vi "Configure Instrument.vi"(8 "error in (no error)":errorcluster, 11 "Instrument.Aerotech":refnum<class "Instrument.Aerotech.lvclass">) -> (0 "error out":errorcluster, 3 "Instrument.Aerotech out":refnum<class "Instrument.Aerotech.lvclass">)   [LabVIEW 2016, in "Instrument.Aerotech.lvclass"]
uses:
  Instrument.Aerotech.lvclass
  <userlib>/LevyLab/Levylab Instruments/Instrument Types/Optical Delay Line/Instrument.OpticalDelayLine.lvclass
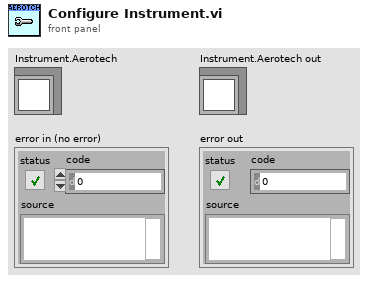
[diagram p1: front panel]
types:
  T1 = typedef "Instrument.Aerotech.lvclass/Instrument.Aerotech.Configuration--Cluster.ctl" = cluster{"Example Setting 1":dbl, "Example Setting 2":dbl, "Example Setting 3":string}
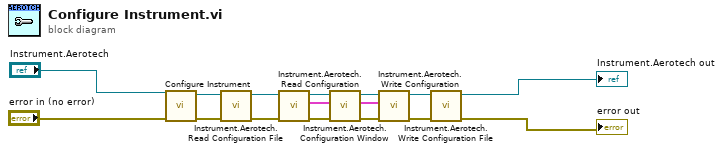
[diagram p0: block diagram]
diagram:
  n1 = call-parent "Configure Instrument.vi"("error in (no error)"="error in (no error)", "Instrument in"="Instrument.Aerotech") -> ("error out"=w11:errorcluster, "Instrument out"=w13:refnum<class "Instrument.Aerotech.lvclass">)  [unwired: 8 in]
  n2 = call "Instrument.Aerotech.Read Configuration File.vi"("error in (no error)"=w11, "Instrument.Aerotech"=w13) -> ("error out"=w10:errorcluster, "Instrument.Aerotech out"=w9:refnum<class "Instrument.Aerotech.lvclass">)  [unwired: 8 in]
  n3 = call "Instrument.Aerotech.Read Configuration.vi"("error in (no error)"=w10, "Instrument.Aerotech"=w9) -> ("error out"=w7:errorcluster, "Configuration"=w2:T1, "Instrument.Aerotech out"=w8:refnum<class "Instrument.Aerotech.lvclass">)  [unwired: 7 in]
  n4 = call "Instrument.Aerotech.Configuration Window.vi"("error in (no error)"=w7, "Ex Configuration"=w2, "Instrument.Aerotech"=w8) -> ("error out"=w6:errorcluster, "output cluster"=w1:T1, "Instrument.Aerotech out"=w5:refnum<class "Instrument.Aerotech.lvclass">)  [unwired: 6 in]
  n5 = call "Instrument.Aerotech.Write Configuration.vi"("error in (no error)"=w6, "Configuration"=w1, "Instrument.Aerotech"=w5) -> ("error out"=w3:errorcluster, "Instrument.Aerotech out"=w4:refnum<class "Instrument.Aerotech.lvclass">)  [unwired: 7 in]
  n6 = call "Instrument.Aerotech.Write Configuration File.vi"("error in (no error)"=w3, "Instrument.Aerotech"=w4) -> ("error out"=→"error out":errorcluster, "Instrument.Aerotech out"=→"Instrument.Aerotech out":refnum<class "Instrument.Aerotech.lvclass">)  [unwired: 8 in]
